vi "Pong.vi"(8 "error in (no error)":errorcluster, 9 "timeout ms (5000)":i32=5000, 10 "Ping Payload":u8[](array[numeric]), 11 "WebSocket in":refnum<class "WebSocket.lvclass">) -> (0 "error out":errorcluster, 1 "timed out?":bool, 3 "WebSocket out":refnum<class "WebSocket.lvclass">)   [LabVIEW 2021, in "WebSockets.lvlib" / "WebSocket.lvclass"]
doc: "Sends a Pong frame to the connection endpoint, the payload should contain the payload from the received Ping request.\nWebSockets 2.0.1.40\nSam Sharp - MediaMongrels Ltd\nCopyright (c) 2019, MediaMongrels Ltd"
uses:
  WebSocket.lvclass
  Opcodes.ctl
  WebSocket.lvclass/WebSocket.ctl
  DataLengthBytes.vi
  EncodeMaskedBytes.vi
  Socket Write.vi
  Sockets/Socket/Socket.lvclass
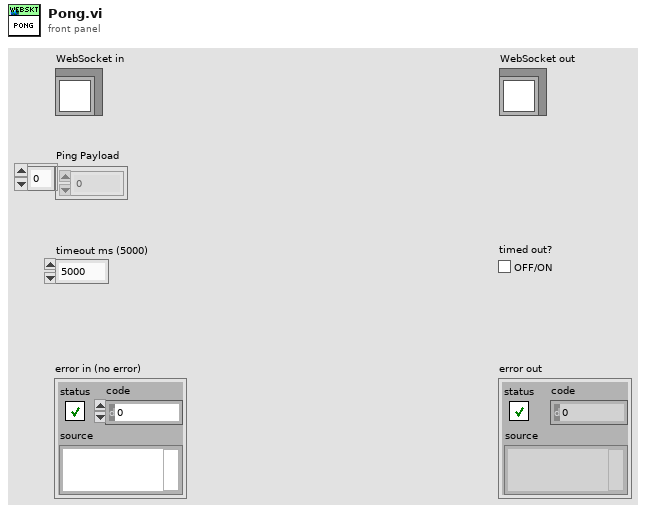
[diagram p1: front panel]
types:
  T1 = typedef "WebSockets.lvlib/WebSocket.lvclass/Opcodes.ctl" = u8
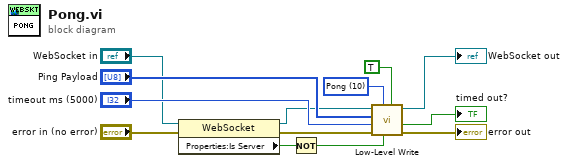
[diagram p0: block diagram]
diagram:
  w7 = T1 10 items=["Cont. Frame"=0, "Text"=1, "Binary"=2, "Close Frame"=8, "Ping"=9, "Pong"=10] ("Opcode (Text)")
  n1 = property class="WebSocket"(reference="WebSocket in", error in="error in (no error)") -> (reference out=w4:refnum<class "WebSocket.lvclass">, error out=w6:errorcluster, "Properties:Is Server"=w3:bool)
  n2 = Not(x=w3) -> (.not. x?=w2:bool)
  n3 = call "Low-Level Write.vi"("Finished? (True)"=TRUE, "Mask payload?"=w2, "Opcode (Text)"=w7, "error in (no error)"=w6, "timeout ms (5000)"="timeout ms (5000)", "Data"="Ping Payload", "WebSockets in"=w4) -> ("error out"=→"error out":errorcluster, "timed out?"=→"timed out?":bool, "WebSockets out"=→"WebSocket out":refnum<class "WebSocket.lvclass">)  [unwired: 2 in]
